vi "Throttle Driver.vi"(8 "Reference Voltage In":fxp<+/-,24,5>=5.0, 9 "Throttle Max":fxp<+,16,4>, 10 "Throttle Min":fxp<+,16,4>, 11 "Throttle Voltage In":fxp<+/-,26,5>=5.0) -> (0 "Unscaled Throttle Percent":fxp<+/-,16,1>, 2 "Throttle Percent":fxp<+/-,27,18>, 3 "In Range":bool)   [LabVIEW 2015]
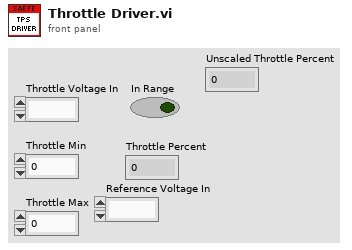
[diagram p1: front panel]
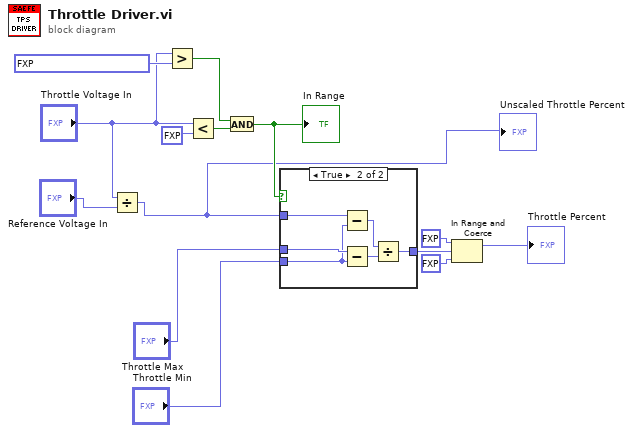
[diagram p0: block diagram]
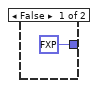
[diagram p2: hidden frame]
diagram:
  n1 = Divide(x="Throttle Voltage In", y="Reference Voltage In") -> (x/y=w1:fxp<+/-,16,1>)
  "Unscaled Throttle Percent" <- w1
  n2 = Greater?(x="Throttle Voltage In", y=fxp<+/-,26,5> 0.19999980926513672) -> (0:w11:bool)
  n3 = Less?(x="Throttle Voltage In", y=fxp<+/-,26,5> 4.5) -> (x < y?=w12:bool)
  n4 = And(x=w11, y=w12) -> (x .and. y?=w14:bool)
  "In Range" <- w14
  n5 = case shown="True" w14 {
    tunnel: w1 -> [_ w21]
    tunnel: "Throttle Min" -> [_ w18]
    tunnel: "Throttle Max" -> [_ w19]
    tunnel: [fxp<+/-,27,18> 0.0 w16] -> w7
    frame False {
    }
    frame True {
      n6 = Subtract(x=w21, y=w18) -> (x-y=w20:fxp<+/-,21,6>)
      n7 = Subtract(x=w19, y=w18) -> (x-y=w17:fxp<+/-,17,5>)
      n8 = Divide(x=w20, y=w17) -> (x/y=w16:fxp<+/-,27,18>)
    }
  }
  n9 = In Range and Coerce(upper limit=fxp<+/-,27,18> 1.0, x=w7, lower limit=fxp<+/-,27,18> 0.0) -> (coerced(x)=→"Throttle Percent":fxp<+/-,27,18>)  [unwired: 1 out]
